vi "Pressure_Multiplexer_Remote.vi"() -> (0 "DAQ Error":errorcluster)   [LabVIEW 2021]
uses:
  Globals/Meas_global.vi
  Sub_vis/Upload Data.ctl
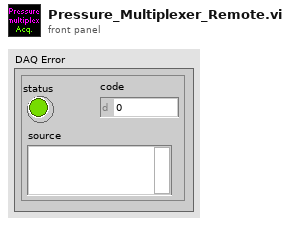
[diagram p1: front panel]
types:
  T1 = typedef "Setup.ctl" = enum16{"Run Program", "Show Setup", "Save Current Setup", "Setup Front Panel"}
  T2 = typedef "Upload Data.ctl" = enum16{"Voltage Array", "Time Trace Cluster"}
  T3 = typedef "Analysis_info_cluster.ctl" = cluster{"Colour":u32, "Inst type":T4, "Inst name":string, "Symbol":string, "Code name":string, "Extra Info":string, "Inst Array":T5, "Extra Titles":string[], "Extra Values":string[], "U":dbl, "u^2":dbl, "u^3":dbl, "u^4":dbl, "Skew_u":dbl, "Kurt_u":dbl, "Sd Error in Mean":dbl, "% u'/U":dbl, "X":dbl, "Y":dbl, "Z":dbl, "Timescale integral Estimate":dbl, "Sd Error in Variance":dbl, "Calib File":path, "Calib Constants":dbl[], "Output Position":bool, "Stats":enum16{"None", "Basic", "Full"}, "Av Sampling Rate":dbl, "Av No of Samples":dbl, "Total Meas Time (s)":dbl, "ADAM Ch Name":string, "Max value":dbl, "Min value":dbl, "Req Sample Rate Hz":dbl, "Sync Delay Time (s)":dbl, "Ch No":i16, "Device":string, "Use Latest Calib":bool, "Port":string, "Metadata Ch Names":string[], "Metadata Ch Values":string[], "Label":string}
  T4 = typedef "Inst_type.ctl" = enum16{"Raw voltage", "Raw with zero offsetting", "Propeller anemometer", "Pressure Transducer", "Pitot-static tube", "Hot wire", "Cross wire 1", "Cross wire 2", "Generic Linear", "Generic Polynomial", "Generic BackPoly", "Fast FID", "Thermocouple", "Cold wire", "Pulsed Wire", "LDA Vel", "LDA Tran time", "LDA Arr time", "Microphone"}
  T5 = typedef "Instrument_Array.ctl" = enum16{"PWA", "LDA", "Analogue"}
  T6 = typedef "Device ID port info.ctl" = cluster{"Ch No":i16[], "Req Sampling Rate":dbl[], "Port":string, "Index":i32[]}
  T7 = typedef "Rendezvous RefNum" = refnum<k1>
  T8 = typedef "Time_Trace_Cluster.ctl" = cluster{"Weighting":dbl[], "Voltage":dbl[], "Eng Values":dbl[]}
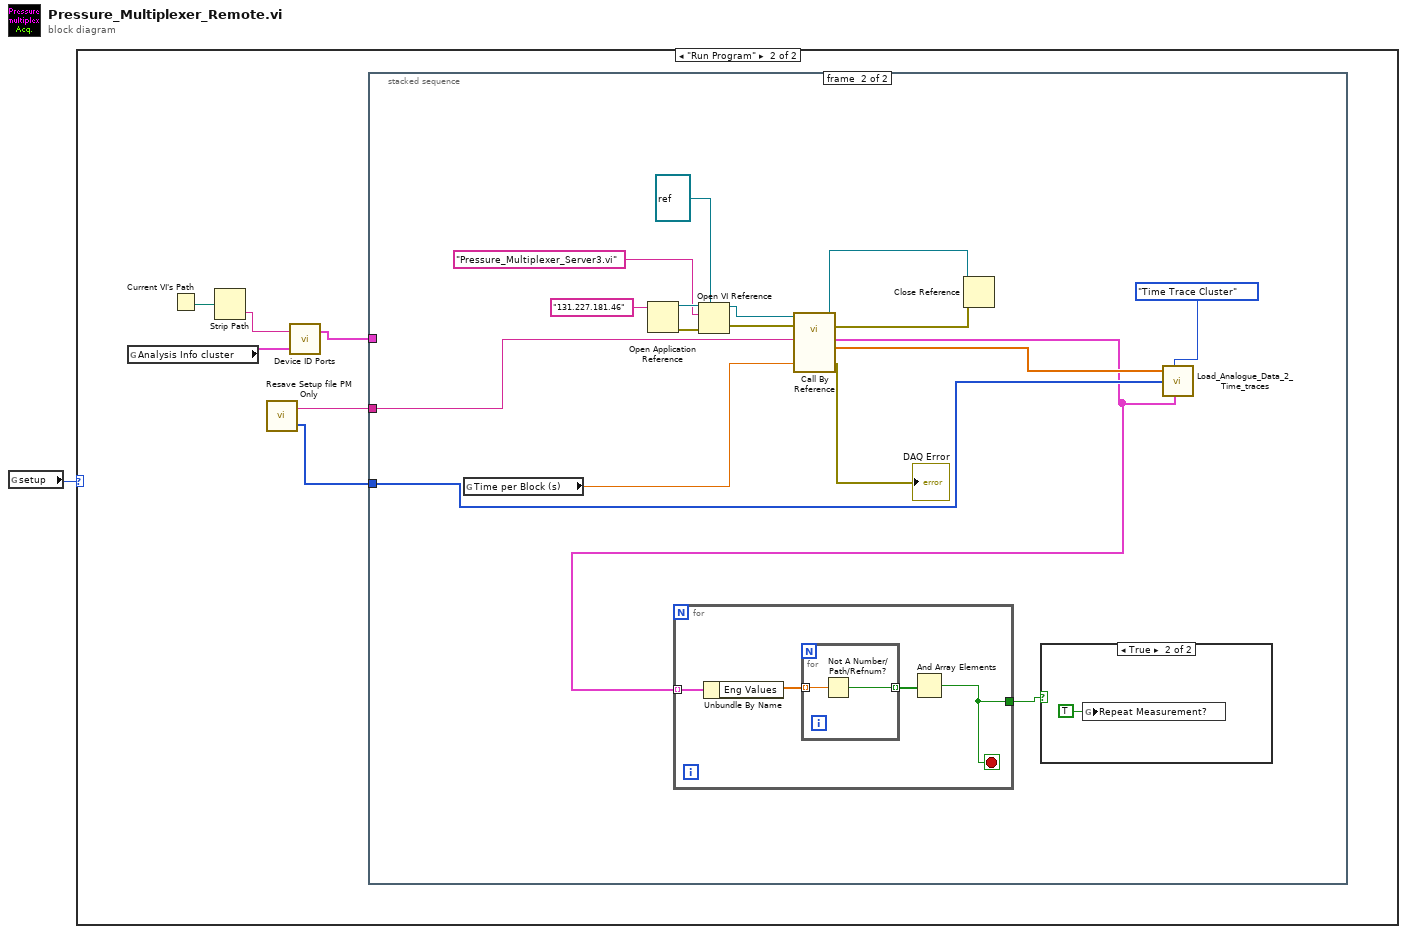
[diagram p0: block diagram]
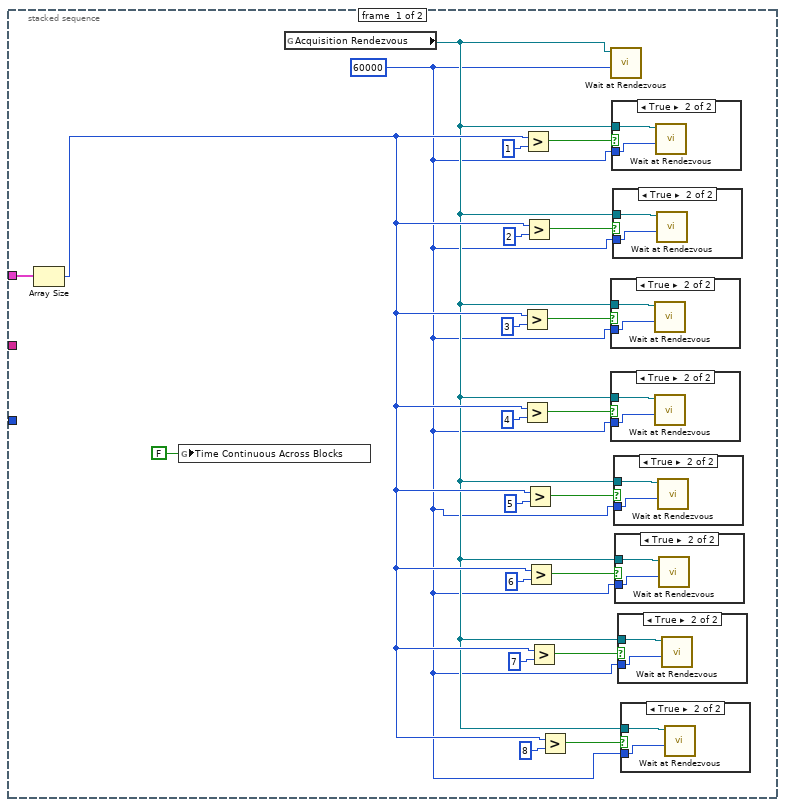
[diagram p3: hidden frame]
diagram:
  n1 = global read "Meas_global.vi" "setup"() -> (w1:T1)
  n2 = case shown="\"Run Program\"" w1 {
    frame Default {
    }
    frame "Run Program" {
      n3 = global read "Meas_global.vi" "Analysis Info cluster"() -> (w7:T3[])
      n4 = Current VI's Path() -> (path=w5:path)
      n5 = Strip Path(path=w5) -> (name=w6:string)  [unwired: 1 out]
      n6 = call "Resave Setup file PM Only.vi"() -> ("PM index"=w2:i32[], "Setup filename"=w3:string)  [unwired: 2 in]
      n7 = call "Device ID Ports.vi"("Analysis Info cluster"=w7, "Device ID"=w6) -> ("Device port info"=w4:T6[])  [unwired: 1 out]
      n8 = stacked-sequence {
        tunnel: w4 -> [w26 _]
        tunnel: w3 -> [_ w50]
        tunnel: w2 -> [_ w48]
        frame #0 {
          w8 = 60000 ("ms timeout (-1)")
          n9 = Array Size(array=w26) -> (size(s)=w27:i32)
          n10 = global write "Meas_global.vi" "Time Continuous Across Blocks"(FALSE ("Time Continuous across Blocks")) -> ()
          n11 = global read "Meas_global.vi" "Acquisition Rendezvous"() -> (w10:T7)
          n12 = Greater?(x=w27, y=3) -> (0:w16:bool)
          n13 = Greater?(x=w27, y=4) -> (0:w15:bool)
          n14 = Greater?(x=w27, y=1) -> (0:w18:bool)
          n15 = Greater?(x=w27, y=2) -> (0:w17:bool)
          n16 = Greater?(x=w27, y=5) -> (0:w14:bool)
          n17 = Greater?(x=w27, y=6) -> (0:w13:bool)
          n18 = Greater?(x=w27, y=7) -> (0:w12:bool)
          n19 = Greater?(x=w27, y=8) -> (0:w9:bool)
          n20 = call <vilib>:"Wait at Rendezvous.vi"("ms timeout (-1)"=w8, "rendezvous"=w10) -> ()  [unwired: 3 in, 3 out]
          n21 = case shown="True" w16 {
            tunnel: w10 -> [_ w34]
            tunnel: w8 -> [_ w33]
            frame False {
            }
            frame True {
              n22 = call <vilib>:"Wait at Rendezvous.vi"("ms timeout (-1)"=w33, "rendezvous"=w34) -> ()  [unwired: 3 in, 3 out]
            }
          }
          n23 = case shown="True" w15 {
            tunnel: w10 -> [_ w36]
            tunnel: w8 -> [_ w35]
            frame False {
            }
            frame True {
              n24 = call <vilib>:"Wait at Rendezvous.vi"("ms timeout (-1)"=w35, "rendezvous"=w36) -> ()  [unwired: 3 in, 3 out]
            }
          }
          n25 = case shown="True" w18 {
            tunnel: w10 -> [_ w44]
            tunnel: w8 -> [_ w43]
            frame False {
            }
            frame True {
              n26 = call <vilib>:"Wait at Rendezvous.vi"("ms timeout (-1)"=w43, "rendezvous"=w44) -> ()  [unwired: 3 in, 3 out]
            }
          }
          n27 = case shown="True" w17 {
            tunnel: w10 -> [_ w32]
            tunnel: w8 -> [_ w31]
            frame False {
            }
            frame True {
              n28 = call <vilib>:"Wait at Rendezvous.vi"("ms timeout (-1)"=w31, "rendezvous"=w32) -> ()  [unwired: 3 in, 3 out]
            }
          }
          n29 = case shown="True" w14 {
            tunnel: w10 -> [_ w38]
            tunnel: w8 -> [_ w37]
            frame False {
            }
            frame True {
              n30 = call <vilib>:"Wait at Rendezvous.vi"("ms timeout (-1)"=w37, "rendezvous"=w38) -> ()  [unwired: 3 in, 3 out]
            }
          }
          n31 = case shown="True" w13 {
            tunnel: w10 -> [_ w40]
            tunnel: w8 -> [_ w39]
            frame False {
            }
            frame True {
              n32 = call <vilib>:"Wait at Rendezvous.vi"("ms timeout (-1)"=w39, "rendezvous"=w40) -> ()  [unwired: 3 in, 3 out]
            }
          }
          n33 = case shown="True" w12 {
            tunnel: w10 -> [_ w42]
            tunnel: w8 -> [_ w41]
            frame False {
            }
            frame True {
              n34 = call <vilib>:"Wait at Rendezvous.vi"("ms timeout (-1)"=w41, "rendezvous"=w42) -> ()  [unwired: 3 in, 3 out]
            }
          }
          n35 = case shown="True" w9 {
            tunnel: w10 -> [_ w30]
            tunnel: w8 -> [_ w29]
            frame False {
            }
            frame True {
              n36 = call <vilib>:"Wait at Rendezvous.vi"("ms timeout (-1)"=w29, "rendezvous"=w30) -> ()  [unwired: 3 in, 3 out]
            }
          }
        }
        frame #1 {
          n37 = global read "Meas_global.vi" "Time per Block (s)"() -> (w55:dbl)
          n38 = Open Application Reference(11:"131.227.181.46" ("machine name (\"\":  open local reference)")) -> (0:w60:errorcluster, 3:w61:refnum<vi>)  [unwired: 2 in, 1 out]
          n39 = Open VI Reference(type specifier VI Refnum (for type only)=refnum<vi> refnum ("Scout Server"), application reference (local)=w61, vi path="Pressure_Multiplexer_Server3.vi", error in (no error)=w60) -> (vi reference=w57:refnum<vi>, error out=w56:errorcluster)  [unwired: 2 out]
          n40 = call-by-ref "?"(reference=w57, error in=w56, "Time per Block (s)"=w55, "Setup filename"=w50) -> (reference out=w54:refnum<vi>, error out=w53:errorcluster, "DAQ Error"=→"DAQ Error":errorcluster, "Av Sampling Rate"=w47:dbl[], "Time Trace"=w46:T8[])  [unwired: 7 in]
          n41 = for {
            tunnel: w46 -> [w66] mode=indexing
            tunnel: [w63] -> w45
            stop <- w63 stop-if-true
            n42 = Unbundle By Name(w66) -> ("Eng Values"=w65:dbl[])
            n43 = for {
              tunnel: w65 -> [w68] mode=indexing
              tunnel: [w67] -> w64 mode=indexing
              n44 = Not A Number/Path/Refnum?(number/path/refnum=w68) -> (NaN/Path/Refnum?=w67:bool)
            }
            n45 = And Array Elements(Boolean array=w64) -> (logical AND=w63:bool)
          }
          n46 = Close Reference(reference=w54, error in (no error)=w53) -> ()  [unwired: 1 out]
          n47 = case shown="True" w45 {
            frame False {
            }
            frame True {
              n48 = global write "Meas_global.vi" "Repeat Measurement?"(TRUE ("Repeat Measurement?")) -> ()
            }
          }
          n49 = call "Load_Analogue_Data_2_Time_traces.vi"("Sampling Rate (Hz)"=w47, "Mode"=Upload_Data."Time Trace Cluster", "Index"=w48, "Time Trace"=w46) -> ()  [unwired: 3 in]
        }
      }
    }
  }
